vi "Analog Input - Voltage and Thermocouple in a Single Task.vi"() -> ()   [LabVIEW 2021]
doc: "This example demonstrates how to continuously acquire buffered voltage and thermocouple measurements using a DAQmx device via a single task. In general, DAQmx Create Channel.vi may be called multiple times within a single analog input task if you need to use different channel settings (measurement types, ranges, etc.) across channels on a single device.\n\nFor instructions on how to connect your signals to the DAQ device, refer to your device documentation."
uses:
  <vilib>/Utility/error.llb/DialogType.ctl
  <vilib>/DAQmx/read.llb/DAQmx Read (Analog 1D Wfm NChan NSamp).vi
  <vilib>/DAQmx/create/channels.llb/DAQmx Create Channel (AI-Voltage-Basic).vi
  <vilib>/DAQmx/create/channels.llb/DAQmx Create Channel (AI-Temperature-Thermocouple).vi
  <vilib>/DAQmx/configure/timing.llb/DAQmx Timing (Sample Clock).vi
  <vilib>/DAQmx/configure/task.llb/DAQmx Configure Logging (TDMS).vi
  <vilib>/DAQmx/miscellaneous.llb/DAQmx Fill In Error Info.vi
  <resource>/objmgr/daqmx.rc
panel:
  in  "Stop":bool
  in  "Channel Settings":enum32{"Voltage", "Thermocouple"}(tab)
  in  "Terminal Configuration":i32(ring)=-1 items=["default"=-1, "RSE"=10083, "NRSE"=10078, "Differential"=10106, "Pseudodifferential"=12529]
  in  "Voltage Physical Channels":tag="PXI2Slot2/ai0" caption="Physical Channels"
  in  "Voltage Min Value":dbl=-5.0 caption="Min Value"
  in  "Voltage Max Value":dbl=5.0 caption="Max Value"
  in  "Enable Voltage":bool=TRUE
  in  "Thermocouple Physical Channels":tag="PXI2Slot2/ai1" caption="Physical Channels"
  in  "Thermocouple Min Value":dbl caption="Min Value"
  in  "Thermocouple Max Value":dbl=100.0 caption="Max Value"
  in  "Units":i32(ring)=10143 items=["Deg C"=10143, "Deg F"=10144, "Kelvins"=10325, "Deg R"=10145, "From Custom Scale"=10065]
  in  "Thermocouple Type":i32(ring)=10072 items=["J"=10072, "K"=10073, "N"=10077, "R"=10082, "S"=10085, "T"=10086, "B"=10047, "E"=10055]
  in  "CJC Source":i32(ring)=10116 items=["Built-In"=10200, "Constant Value"=10116, "Channel"=10113]
  in  "CJC Value":dbl=25.0
  in  "CJC Channel":refnum<k21>
  in  "Enable Thermocouple":bool=TRUE
  in  "TDMS File Path":path
  in  "Logging Mode":i32(ring)=10231 items=["Off"=10231, "Log and Read"=15842]
  in  "Samples per Loop":i32=1000
  in  "Sample Rate":dbl=1000.0
  in  "Sample Clock Source":tag="OnboardClock"
  out "Actual Sample Rate":dbl=1000.0 format="%0.2f"
  out "Waveform Graph":waveform(dbl)[](graph)
  # "Channel Settings"
  # "Timing Settings"
  # "Logging Settings"
  # "Acquired Data"
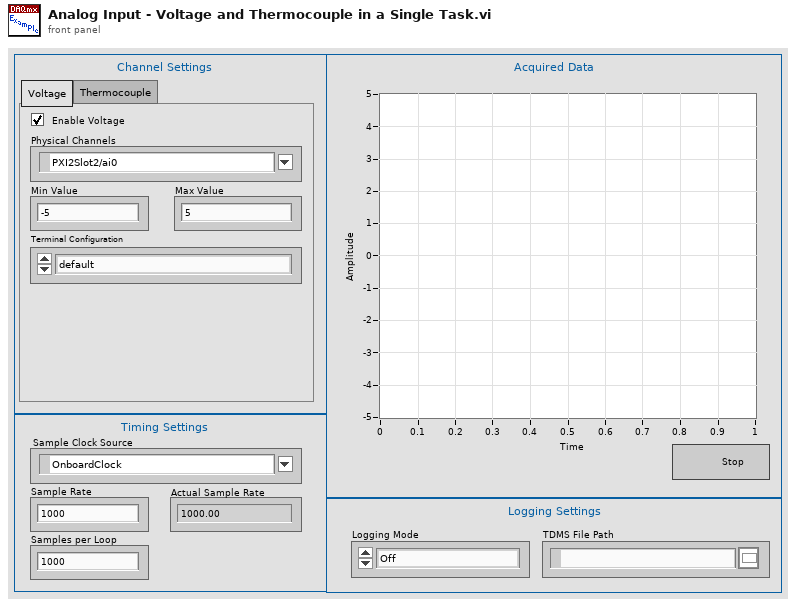
[diagram p1: front panel]
types:
  T1 = typedef "DialogType.ctl" = u16
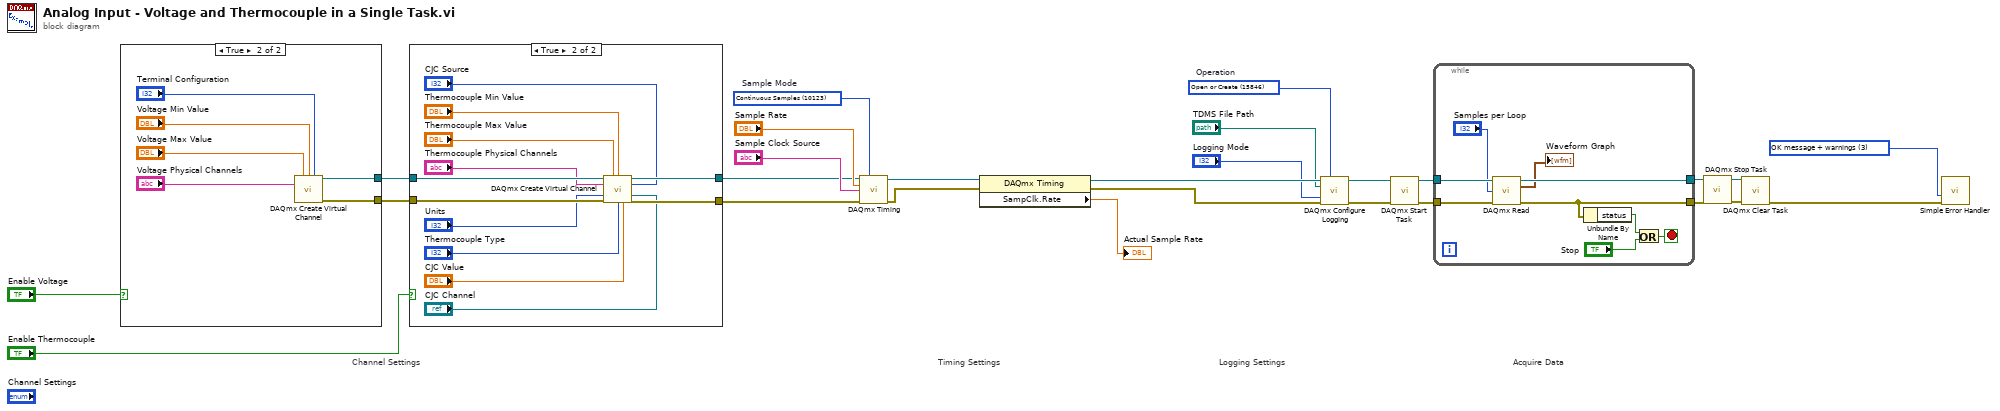
[diagram p0: block diagram]
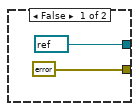
[diagram p3: hidden frame]
diagram:
  w1 = T1 3 items=["no dialog", "OK message", "continue or stop message", "OK message + warnings", "continue/stop + warnings"] ("type of dialog (OK msg:1)")
  w22 = 15846 items=["Open"=10437, "Open or Create"=15846, "Create or Replace"=15847, "Create"=15848]  # Operation
  w25 = 10123 items=["Finite Samples"=10178, "Continuous Samples"=10123, "Hardware Timed Single Point"=12522]  # Sample Mode
  # "Acquire Data"
  # "Timing Settings"
  # "Channel Settings"
  # "Logging Settings"
  n1 = case shown="True" "Enable Voltage" {
    tunnel: [errorcluster {"status"=FALSE, "code"=0, "source"=""} ("error out") w35] -> w11
    tunnel: [refnum<k21> refnum ("task out") w34] -> w10
    frame False {
    }
    frame True {
      n2 = call-poly <vilib>:"DAQmx Create Virtual Channel.vi"("maximum value"="Voltage Max Value", "minimum value"="Voltage Min Value", "input terminal configuration"="Terminal Configuration", "physical channels"="Voltage Physical Channels") -> ("task out"=w34:refnum<k21>, "error out"=w35:errorcluster)  [unwired: 10 in]
    }
  }
  n3 = case shown="True" "Enable Thermocouple" {
    tunnel: [w36 w49] -> w8
    tunnel: [w37 w48] -> w9
    tunnel: w11 -> [w36 w47]
    tunnel: w10 -> [w37 w46]
    frame False {
    }
    frame True {
      n4 = call-poly <vilib>:"DAQmx Create Virtual Channel.vi"("task in"=w46, "maximum value"="Thermocouple Max Value", "minimum value"="Thermocouple Min Value", "physical channels"="Thermocouple Physical Channels", "cjc source"="CJC Source", "units"="Units", "cjc channel"="CJC Channel", "error in"=w47, "thermocouple type"="Thermocouple Type", "cjc value"="CJC Value") -> ("task out"=w48:refnum<k21>, "error out"=w49:errorcluster)  [unwired: 4 in]
    }
  }
  n5 = call-poly <vilib>:"DAQmx Timing.vi"("task/channels in"=w9, "sample mode"=w25, "rate"="Sample Rate", "source"="Sample Clock Source", "error in"=w8) -> ("task out"=w27:refnum<k21>, "error out"=w26:errorcluster)  [unwired: 9 in]
  n6 = property class="DAQmx Timing"(reference=w27, error in=w26) -> (reference out=w24:refnum<k21>, error out=w23:errorcluster, "SampClk.Rate"=→"Actual Sample Rate":dbl)
  n7 = call-poly <vilib>:"DAQmx Configure Logging.vi"("task/channels in"=w24, "operation"=w22, "file path"="TDMS File Path", "logging mode"="Logging Mode", "error in"=w23) -> ("task out"=w13:refnum<k21>, "error out"=w12:errorcluster)  [unwired: 9 in]
  n8 = call <vilib>:"DAQmx Start Task.vi"("task/channels in"=w13, "error in"=w12) -> ("task out"=w21:refnum<k21>, "error out"=w20:errorcluster)  [unwired: 12 in]
  n9 = while {
    tunnel: w21 -> [w58]
    tunnel: w20 -> [w57]
    tunnel: [w54] -> w2
    tunnel: [w55] -> w3
    stop <- w56 stop-if-true
    n10 = call-poly <vilib>:"DAQmx Read.vi"("task/channels in"=w58, "number of samples per channel"="Samples per Loop", "error in"=w57) -> ("task out"=w55:refnum<k21>, "data"=→"Waveform Graph":waveform(dbl)[], "error out"=w54:errorcluster)  [unwired: 10 in]
    n11 = Unbundle By Name(w54) -> ("status"=w53:bool)
    n12 = Or(x=w53, y="Stop") -> (x .or. y?=w56:bool)
  }
  n13 = call <vilib>:"DAQmx Stop Task.vi"("task/channels in"=w3, "error in"=w2) -> ("task out"=w5:refnum<k21>, "error out"=w4:errorcluster)  [unwired: 12 in]
  n14 = call <vilib>:"DAQmx Clear Task.vi"("task in"=w5, "error in"=w4) -> ("error out"=w19:errorcluster)  [unwired: 13 in]
  n15 = call <vilib>:"Simple Error Handler.vi"("type of dialog (OK msg:1)"=w1, "error in (no error)"=w19) -> ()  [unwired: 3 in, 5 out]
